vi "Lithography Legacy Convert_MFP3D.vi"(1 "Amplifier Setting":dbl=-15.0, 2 "Lithography Data":T1(array[cluster])) -> (0 "Array":T2(array[cluster]))   [LabVIEW 2016]
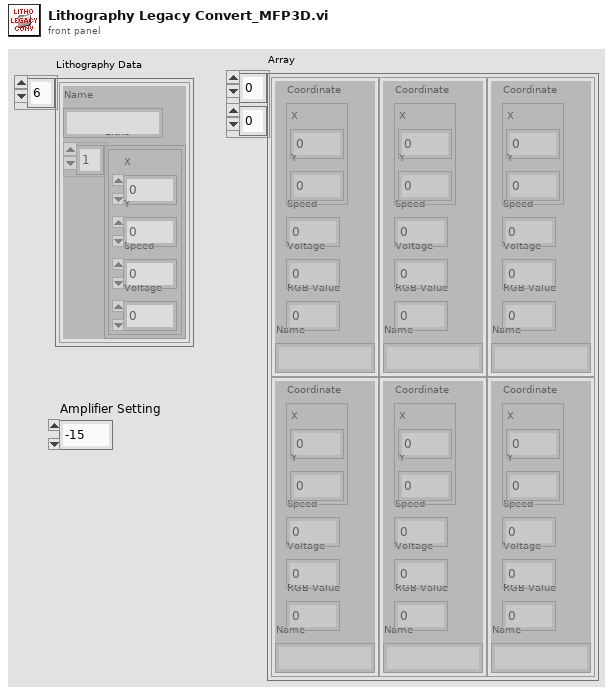
[diagram p1: front panel]
types:
  T1 = cluster{"Name":string, "Litho":cluster{"X":dbl, "Y":dbl, "Speed":dbl, "Voltage":dbl}[]}[]
  T2 = cluster{"Coordinate":cluster{"X":dbl, "Y":dbl}, "Speed":dbl, "Voltage":dbl, "RGB Value":dbl, "Name":string}[][]
  T3 = cluster{"Coordinate":cluster{"X":dbl, "Y":dbl}, "Speed":dbl, dbl, "Voltage":dbl, "Name":string}[][]
  T4 = cluster{"X":dbl, "Y":dbl, "Speed":dbl, "Voltage":dbl}[]
  T5 = cluster{"Coordinate":cluster{"X":dbl, "Y":dbl}, "Speed":dbl, dbl, "Voltage":dbl, "Name":string}
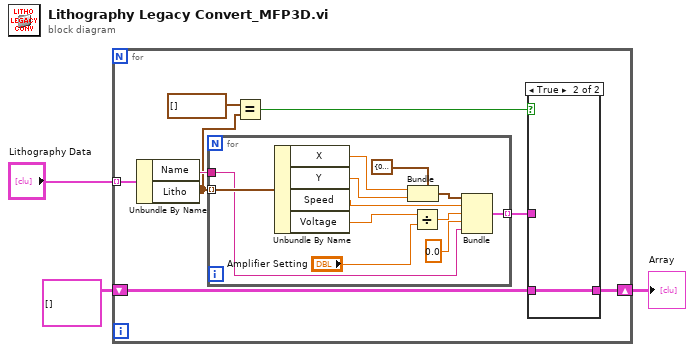
[diagram p0: block diagram]
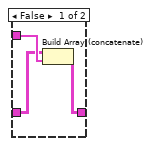
[diagram p2: hidden frame]
diagram:
  n1 = for {
    tunnel: "Lithography Data" -> [w11] mode=indexing
    shift-right: [w9] -> w1
    shift-left: T3 [] -> [w8]
    n2 = Unbundle By Name(w11) -> ("Name"=w10:string, "Litho"=w4:T4)
    n3 = for {
      tunnel: w4 -> [w27] mode=indexing
      tunnel: w10 -> [w21]
      tunnel: [w20] -> w7 mode=indexing
      n4 = Unbundle By Name(w27) -> ("X"=w26:dbl, "Y"=w25:dbl, "Speed"=w22:dbl, "Voltage"=w18:dbl)
      n5 = Bundle(cluster=cluster{"X":dbl, "Y":dbl} {"X"=0.0, "Y"=0.0} ("Coordinate"), "X"=w26, "Y"=w25) -> (w23:cluster{"X":dbl, "Y":dbl})
      n6 = Divide(x=w18, y="Amplifier Setting") -> (x/y=w17:dbl)
      n7 = Bundle("Coordinate"=w23, "Speed"=w22, w17, "Voltage"=0.0, "Name"=w21) -> (w20:T5)  [unwired: 1 in]
    }
    n8 = Equal?(x=T4 [] ("Litho"), y=w4) -> (x = y?=w6:bool)
    n9 = case shown="True" w6 {
      tunnel: [w14 w15] -> w9
      tunnel: w8 -> [w12 w15]
      tunnel: w7 -> [w13 _]
      frame False {
        n10 = Build Array (concatenate)(w12, w13) -> (w14:T3)
      }
      frame True {
      }
    }
  }
  "Array" <- w1
